vi "Create Named Group.vi"(0 "HDF5 Ref":T1, 2 "variant":variant, 3 "error in (no error)":errorcluster) -> (5 "HDF5 Ref out":T1, 6 "HDF5 Group Ref":T1, 7 "variant out":variant, 8 "error out":errorcluster)   [LabVIEW 2019]
uses:
  <vilib>/UPVI/lvhdf5/library.llb/HDF5 Ref.ctl
  <vilib>/UPVI/lvhdf5/group.llb/OpenCreateGroup (String).vi
  <vilib>/Utility/Data Type/NI_Data Type.lvlib
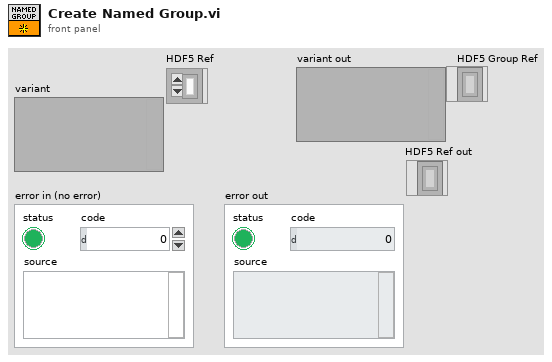
[diagram p1: front panel]
types:
  T1 = typedef "HDF5 Ref.ctl" = refnum<k1>
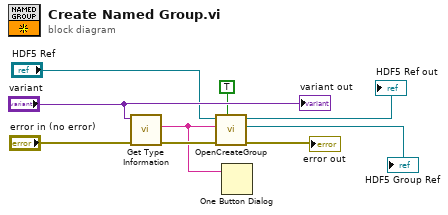
[diagram p0: block diagram]
diagram:
  n1 = call <vilib>:"Get Type Information.vi"("error in (no error)"="error in (no error)", "variant"="variant") -> ("error out"=w7:errorcluster, "name"=w2:string)  [unwired: 5 in, 3 out]
  n2 = call-poly <vilib>:"OpenCreateGroup.vi"("Create if not found (F)"=TRUE, "error in (no error)"=w7, "Group"=w2, "HDF5 Ref"="HDF5 Ref") -> ("error out"=→"error out":errorcluster, "HDF5 Group Ref"=→"HDF5 Group Ref":T1, "HDF5 Ref out"=→"HDF5 Ref out":T1)  [unwired: 5 in]
  n3 = One Button Dialog(message=w2) -> ()  [unwired: 1 in, 1 out]
  "variant out" <- "variant"
